vi "Epoxy_Cycle Time.vi"(7 "Enum":T1, 8 "error in (no error)":errorcluster, 10 "Cycle Interval":dbl, 11 "Run?":bool) -> (0 "error out":errorcluster, 1 "Int Lap [s]":dbl, 2 "Cycle done?":bool, 3 "Running?":bool)   [LabVIEW 2020]
uses:
  controls/CycleTimer.ctl
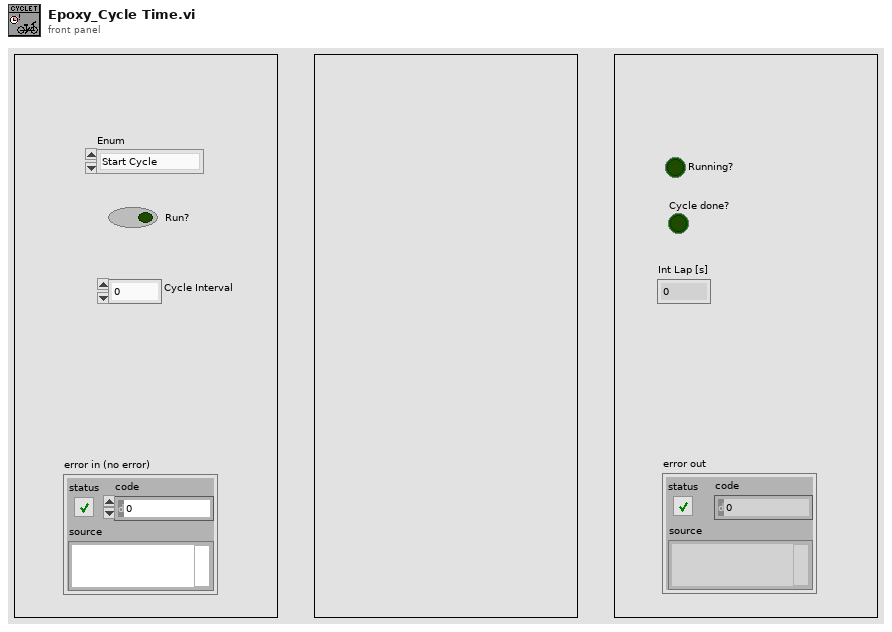
[diagram p1: front panel]
types:
  T1 = typedef "CycleTimer.ctl" = enum16{"Start Cycle", "StartInterval", "UpdateInterval", "Check"}
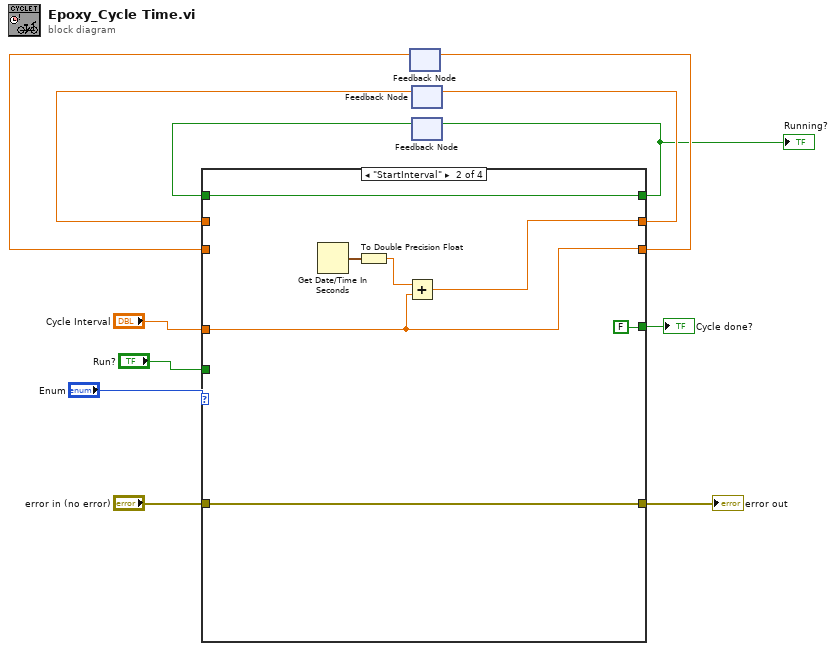
[diagram p0: block diagram]
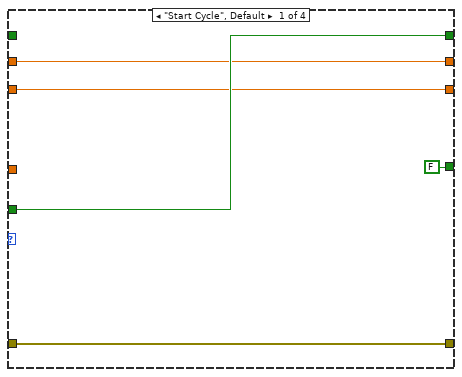
[diagram p2: hidden frame]
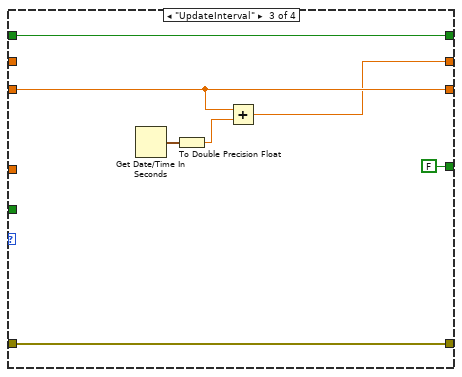
[diagram p3: hidden frame]
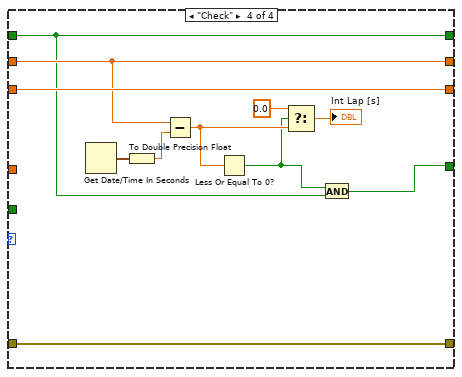
[diagram p4: hidden frame]
diagram:
  n1 = feedback #1() -> (w11:dbl)  [unwired: 1 in]
  n2 = feedback #2() -> (w9:dbl)  [unwired: 1 in]
  n3 = feedback #3() -> (w6:bool)  [unwired: 1 in]
  n4 = case shown="\"StartInterval\"" "Enum" {
    tunnel: "error in (no error)" -> [w17 w24 w31 w42]
    tunnel: [w17 w24 w31 w42] -> w1
    tunnel: "Run?" -> [w16 _ _ _]
    tunnel: [w16 w23 w30 w34] -> w5
    tunnel: w6 -> [_ w23 w30 w34]
    tunnel: "Cycle Interval" -> [_ w19 _ _]
    tunnel: [w14 w20 w26 w39] -> w8
    tunnel: w9 -> [w14 _ _ w39]
    tunnel: [w15 w19 w28 w41] -> w10
    tunnel: w11 -> [w15 _ w28 w41]
    tunnel: [FALSE FALSE FALSE w32] -> w12
    frame "Start Cycle", Default {
    }
    frame "StartInterval" {
      n5 = Get Date/Time In Seconds() -> (seconds since 1Jan1904=w22:timestamp)
      n6 = To Double Precision Float(number=w22) -> (double precision float=w21:dbl)
      n7 = Add(x=w21, y=w19) -> (x+y=w20:dbl)
    }
    frame "UpdateInterval" {
      n8 = Get Date/Time In Seconds() -> (seconds since 1Jan1904=w29:timestamp)
      n9 = To Double Precision Float(number=w29) -> (double precision float=w27:dbl)
      n10 = Add(x=w28, y=w27) -> (x+y=w26:dbl)
    }
    frame "Check" {
      n11 = Get Date/Time In Seconds() -> (seconds since 1Jan1904=w40:timestamp)
      n12 = To Double Precision Float(number=w40) -> (double precision float=w38:dbl)
      n13 = Subtract(x=w39, y=w38) -> (x-y=w36:dbl)
      n14 = Less Or Equal To 0?(x=w36) -> (x <= 0?=w33:bool)
      n15 = Select(t=0.0, s=w33, f=w36) -> (s? t:f=→"Int Lap [s]":dbl)
      n16 = And(x=w33, y=w34) -> (x .and. y?=w32:bool)
    }
  }
  "error out" <- w1
  "Running?" <- w5
  "Cycle done?" <- w12
  n17 = feedback-in #1(w10) -> ()
  n18 = feedback-in #2(w8) -> ()
  n19 = feedback-in #3(w5) -> ()
